vi "getSecondElement_v1.vi"(11 "Input Array":dbl[](array[numeric])) -> (3 "Second Element":dbl)   [LabVIEW 2016]
panel:
  # ">>>"
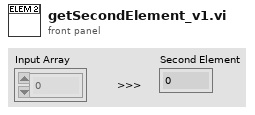
[diagram p1: front panel]
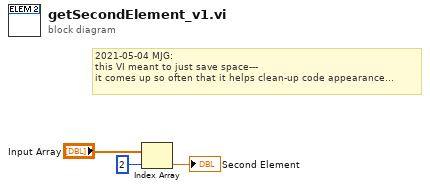
[diagram p0: block diagram]
diagram:
  # "2021-05-04 MJG:\nthis VI meant to just save space---\nit comes up so often that it helps clean-up code appearance..."
  n1 = Index Array(array="Input Array", index=2) -> (element=→"Second Element":dbl)
